vi "Begin.vi"(11 "Image Size":T1=enum."160x120") -> (0 "error out":errorcluster)   [LabVIEW 2012]
doc: "Called before other user functions, this VI is expected to open initial I/O refnums, load in file data, and do all program initialization. Notice that the <B>error out</B> terminal is simply used for data flow. Wiring it to other structures or subVIs ensures that this VI runs first."
uses:
  <vilib>/Rock Robotics/WPI/Camera/WPI_CameraImageSize.ctl
  <vilib>/Rock Robotics/SystemInterfaces/DIO/FPGA_DIOPWMChannel.ctl
  <vilib>/Rock Robotics/WPI/Camera/WPI_CameraWhite Balance Values.ctl
  <vilib>/Rock Robotics/WPI/Camera/WPI_CameraExposure Values.ctl
  <vilib>/Rock Robotics/WPI/Camera/WPI_CameraFrameRate.ctl
  <vilib>/Rock Robotics/WPI/DriverStation/WPI_DriverStationRobotMode2.ctl
  <vilib>/Rock Robotics/WPI/Joystick/WPI_JoystickDeviceEnum.ctl
  <vilib>/Rock Robotics/WPI/SafetyOutput/WPI_SafetyOutputConfigMenu.ctl
  <vilib>/Rock Robotics/WPI/RobotDrive/WPI_RobotDriveOpen2MotorWithJaguar.vi
  Robot Global Data.vi
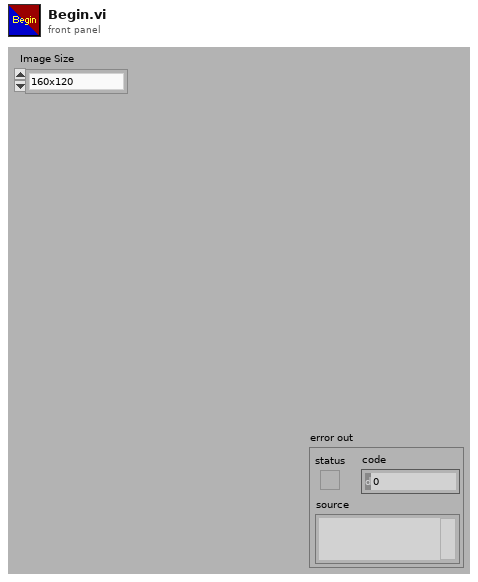
[diagram p1: front panel]
types:
  T1 = typedef "WPI_CameraImageSize.ctl" = enum16{"640x480", "320x240", "160x120"}
  T2 = typedef "WPI_SafetyOutputConfigMenu.ctl" = enum16{"Enable", "Disable"}
  T3 = typedef "FPGA_DIOPWMChannel.ctl" = enum8{"PWM 1", "PWM 2", "PWM 3", "PWM 4", "PWM 5", "PWM 6", "PWM 7", "PWM 8", "PWM 9", "PWM 10", "Invalid"}
  T4 = typedef "WPI_JoystickDeviceEnum.ctl" = enum16{"USB 1", "USB 2", "USB 3", "USB 4", "Kinect 1", "Kinect 2"}
  T5 = typedef "WPI_DriverStationRobotMode2.ctl" = enum16{"Autonomous Disabled", "Autonomous Enabled", "Teleop Disabled", "Teleop Enabled", "Timeout", "Finish", "Test Disabled", "Test Enabled"}
  T6 = typedef "WPI_CameraFrameRate.ctl" = u32
  T7 = typedef "WPI_CameraExposure Values.ctl" = enum16{"Auto", "Flicker-free 50 Hz", "Flicker-free 60 Hz", "Hold current"}
  T8 = typedef "WPI_CameraWhite Balance Values.ctl" = enum16{"Auto", "Fixed indoor", "Fixed outdoor 1", "Fixed outdoor 2", "Fixed fluorescent 1", "Fixed fluorescent 2", "Hold current"}
  T9 = typedef "WPI_RobotDriveDevRef.ctl" = cluster{"DevStatus":errorcluster, "Motors[]":T10[], "Square Inputs":bool, "Max Output":dbl, "Isochronous":bool}
  T10 = typedef "WPI_MotorControlDeviceRef.ctl" = cluster{"DeviceStatus":errorcluster, "Type":enum16{"PWM", "CAN"}, "PWM":cluster{"Digital Module":T11, "PWM Channel":T3, "DeadBand":T12}, "CAN":cluster{"Device Number":u8, "Control Mode":T13, "Semaphore":T14, "Max Vout":dbl}, "Invert":bool, "TransformRef":T15, "InvTransformRef":T15}
  T11 = typedef "FPGA_TypedefDigitalModule.ctl" = enum16{"Digital Module 1", "Digital Module 2"}
  T12 = typedef "WPI_PWMDeadband.ctl" = cluster{"Name":string, "maxPositivePwm":i32, "minPositivePwm":i32, "centerPwm":i32, "maxNegativePwm":i32, "minNegativePwm":i32, "angularRange":u16}
  T13 = typedef "WPI_CANJaguar_ControlMode.ctl" = enum8{"Percent VBus", "Current", "Speed", "Position", "Voltage"}
  T14 = typedef "Semaphore RefNum" = refnum<k1>
  T15 = typedef "WPI_PWMTransform_ConPane.ctl" = refnum<vi>
  T16 = typedef "WPI_CameraDevRef.ctl" = cluster{"Camera Address":string, "CameraStatus":errorcluster, "Acquire Image Notifier":refnum<notifier>}
  T17 = typedef "WPI_JoystickDevRef.ctl" = cluster{"Device":T4}
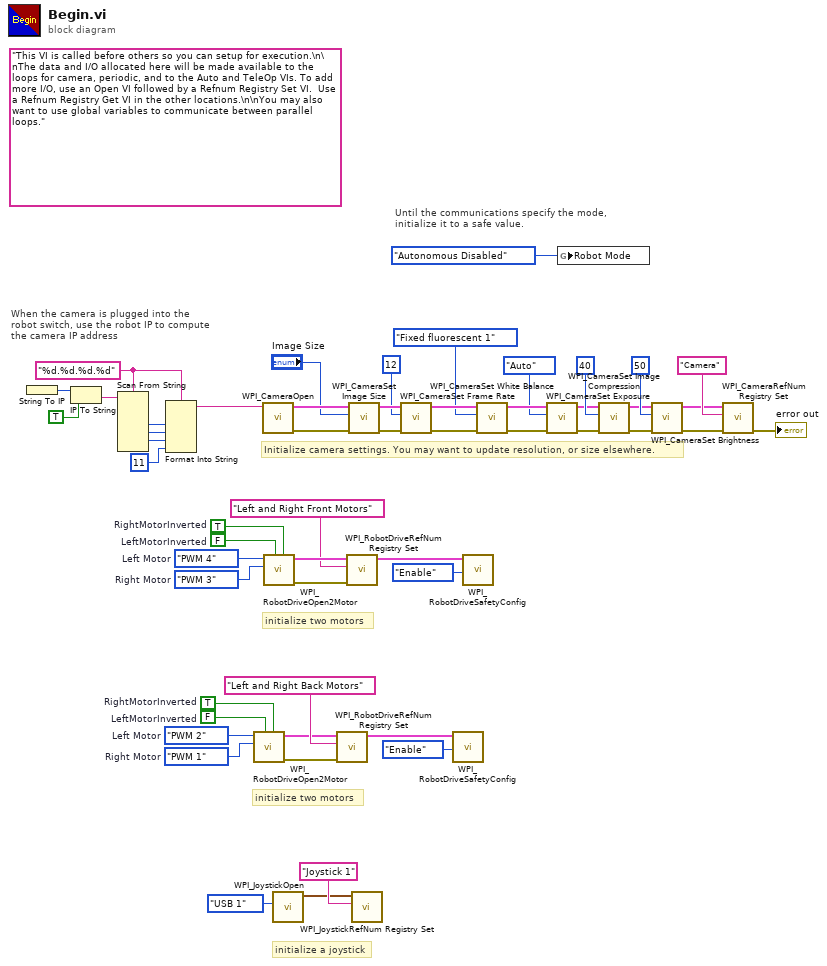
[diagram p0: block diagram]
diagram:
  w7 = FPGA_DIOPWMChannel."PWM 1"  # Right Motor
  w6 = FPGA_DIOPWMChannel."PWM 2"  # Left Motor
  w2 = FALSE  # LeftMotorInverted
  w1 = TRUE  # RightMotorInverted
  w18 = "%d.%d.%d.%d" ("format string")
  (unwired) "This VI is called before others so you can setup for execution.\n\nThe data and I/O allocated here will be made available to the loops for camera, periodic, and to the Auto and TeleOp VIs. To add more I/O, use an Open VI followed by a Refnum Registry Set VI.  Use a Refnum Registry Get VI in the other locations.\n\nYou may also want to use global variables to communicate between parallel loops."
  w29 = FPGA_DIOPWMChannel."PWM 3"  # Right Motor
  w30 = FPGA_DIOPWMChannel."PWM 4"  # Left Motor
  w52 = FALSE  # LeftMotorInverted
  w53 = TRUE  # RightMotorInverted
  # "initialize two motors"
  # "initialize a joystick"
  # "Until the communications specify the mode,\ninitialize it to a safe value."
  # "When the camera is plugged into the\nrobot switch, use the robot IP to compute\nthe camera IP address"
  # "initialize two motors"
  # "Initialize camera settings. You may want to update resolution, or size elsewhere."
  n1 = String To IP() -> (0:w25:u32)  [unwired: 1 in]
  n2 = IP To String(1:TRUE ("dot notation? (F)"), 2:w25) -> (0:w23:string)
  n3 = Scan From String(format string=w18, input string=w23) -> (output 1=w22:i32, output 2=w21:i32, output 3=w20:i32)  [unwired: 7 in, 3 out]
  n4 = Format Into String(format string=w18, w22, w21, w20, 11 ("Compression")) -> (resulting string=w14:string)  [unwired: 2 in, 1 out]
  n5 = call-poly <vilib>:"WPI_RobotDriveOpen2Motor.vi"("Right Motor Inverted"=w1, "Left Motor Inverted"=w2, "Right Motor"=w7, "Left Motor"=w6) -> ("error out"=w5:errorcluster, "RobotDriveDevRef"=w3:T9)  [unwired: 1 in, 5 out]
  n6 = call <vilib>:"WPI_CameraOpen.vi"("Camera Address"=w14) -> ("error out"=w39:errorcluster, "CameraDevRef"=w40:T16)  [unwired: 1 in, 8 out]
  n7 = call-poly <vilib>:"WPI_RobotDriveOpen2Motor.vi"("Right Motor Inverted"=w53, "Left Motor Inverted"=w52, "Right Motor"=w29, "Left Motor"=w30) -> ("error out"=w48:errorcluster, "RobotDriveDevRef"=w50:T9)  [unwired: 1 in, 5 out]
  n8 = call <vilib>:"WPI_JoystickOpen.vi"("JoystickDevice"=WPI_JoystickDeviceEnum."USB 1") -> ("JoystickDevRef"=w12:T17)  [unwired: 10 in]
  n9 = call <vilib>:"WPI_RobotDriveRefNum Registry Set.vi"("error in (no error)"=w5, "refnum name"="Left and Right Back Motors", "RobotDriveDevRef"=w3) -> ("RobotDriveDevRef"=w8:T9)  [unwired: 8 out]
  n10 = call <vilib>:"WPI_RobotDriveRefNum Registry Set.vi"("error in (no error)"=w48, "refnum name"="Left and Right Front Motors", "RobotDriveDevRef"=w50) -> ("RobotDriveDevRef"=w17:T9)  [unwired: 8 out]
  n11 = call <vilib>:"WPI_CameraSet Image Size.vi"("error in (no error)"=w39, "Image Size"="Image Size", "CameraDevRef"=w40) -> ("error out"=w38:errorcluster, "CameraDevRef Out"=w41:T16)  [unwired: 7 out]
  n12 = call <vilib>:"WPI_JoystickRefNum Registry Set.vi"("refnum name"="Joystick 1", "JoystickDevRef"=w12) -> ()  [unwired: 8 in, 2 out]
  n13 = call <vilib>:"WPI_CameraSet Frame Rate.vi"("error in (no error)"=w38, "Frame Rate (fps)"=T6 12, "CameraDevRef"=w41) -> ("error out"=w37:errorcluster, "CameraDevRef Out"=w43:T16)  [unwired: 7 out]
  n14 = call <vilib>:"WPI_RobotDriveSafetyConfig.vi"("mode"=WPI_SafetyOutputConfigMenu."Enable", "RobotDriveDevRef"=w8) -> ()  [unwired: 8 in, 2 out]
  n15 = call <vilib>:"WPI_RobotDriveSafetyConfig.vi"("mode"=WPI_SafetyOutputConfigMenu."Enable", "RobotDriveDevRef"=w17) -> ()  [unwired: 8 in, 2 out]
  n16 = call <vilib>:"WPI_CameraSet White Balance.vi"("error in (no error)"=w37, "White Balance"=WPI_CameraWhite_Balance_Values."Fixed fluorescent 1", "CameraDevRef"=w43) -> ("error out"=w36:errorcluster, "CameraDevRef Out"=w42:T16)  [unwired: 7 out]
  n17 = call <vilib>:"WPI_CameraSet Exposure.vi"("error in (no error)"=w36, "Exposure"=WPI_CameraExposure_Values."Auto", "CameraDevRef"=w42) -> ("error out"=w35:errorcluster, "CameraDevRef Out"=w45:T16)  [unwired: 7 out]
  n18 = global write "Robot Global Data.vi" "Robot Mode"(WPI_DriverStationRobotMode2."Autonomous Disabled" ("Robot Mode")) -> ()
  n19 = call <vilib>:"WPI_CameraSet Image Compression.vi"("error in (no error)"=w35, "Compression"=40, "CameraDevRef"=w45) -> ("error out"=w34:errorcluster, "CameraDevRef Out"=w44:T16)  [unwired: 7 out]
  n20 = call <vilib>:"WPI_CameraSet Brightness.vi"("error in (no error)"=w34, "Brightness"=50, "CameraDevRef"=w44) -> ("error out"=w32:errorcluster, "CameraDevRef Out"=w33:T16)  [unwired: 7 out]
  n21 = call <vilib>:"WPI_CameraRefNum Registry Set.vi"("error in (no error)"=w32, "refnum name"="Camera", "CameraDevRef"=w33) -> ("error out"=→"error out":errorcluster)  [unwired: 8 out]
